vi "DI Read_v1.vi"(8 "error in (no error)":errorcluster, 11 "ControlBoard VISA":refnum<visa-resource-name>="ControlBoard") -> (0 "error out":errorcluster, 1 "DI Reading (Hex String)":string, 2 "DI Reading":bool[](array[boolean]), 3 "VISA Refnum out":refnum<visa-resource-name>)   [LabVIEW 2019]
uses:
  <vilib>/Instr/_visa.llb/VISA Flush IO Buffer Mask.ctl
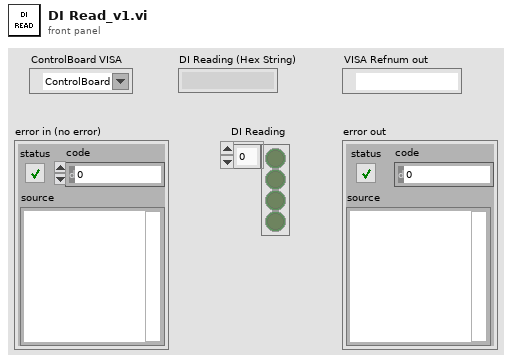
[diagram p1: front panel]
types:
  T1 = typedef "VISA Flush IO Buffer Mask.ctl" = u16
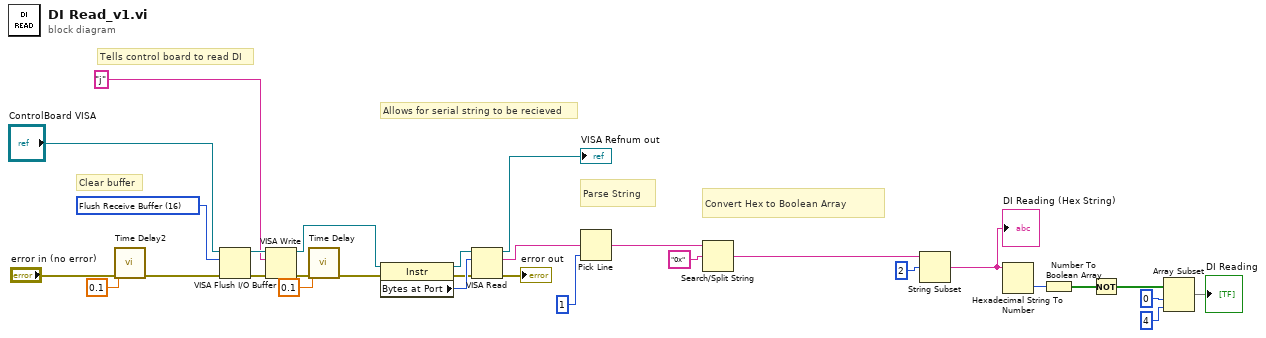
[diagram p0: block diagram]
diagram:
  w19 = T1 16 items=["Flush Receive Buffer"=16, "Write Transmit Buffer to Device"=32, "Flush Receive Buffer (No I/O)"=64, "Flush Transmit Buffer"=128] ("Mask")
  # "Convert Hex to Boolean Array"
  # "Clear buffer"
  # "Parse String"
  # "Allows for serial string to be recieved"
  # "Tells control board to read DI"
  n1 = call "Time Delay2"("error in (no error)"="error in (no error)", "Delay Time (s)"=0.1) -> ("error out"=w5:errorcluster)  [unwired: 9 in]
  n2 = VISA Flush I/O Buffer(VISA resource name="ControlBoard VISA", mask (16)=w19, error in (no error)=w5) -> (VISA resource name out=w21:refnum<visa-resource-name>, error out=w22:errorcluster)
  n3 = VISA Write(VISA resource name=w21, write buffer="j", error in (no error)=w22) -> (VISA resource name out=w24:refnum<visa-resource-name>, error out=w20:errorcluster)  [unwired: 1 out]
  n4 = call "Time Delay"("error in (no error)"=w20, "Delay Time (s)"=0.1) -> ("error out"=w23:errorcluster)  [unwired: 9 in]
  n5 = property class="Instr"(reference=w24, error in=w23) -> (reference out=w16:refnum<visa-resource-name>, error out=w17:errorcluster, "Bytes at Port"=w18:u32)
  n6 = VISA Read(VISA resource name=w16, byte count=w18, error in (no error)=w17) -> (VISA resource name out=→"VISA Refnum out":refnum<visa-resource-name>, read buffer=w28:string, error out=→"error out":errorcluster)  [unwired: 1 out]
  n7 = Pick Line(multi-line string=w28, line index=1) -> (output string=w29:string)  [unwired: 1 in]
  n8 = Search/Split String(string=w29, search string/char (-)="0x" ("regular expression")) -> (match + rest of string=w26:string)  [unwired: 1 in, 2 out]
  n9 = String Subset(string=w26, offset (0)=2) -> (substring=w10:string)  [unwired: 1 in]
  "DI Reading (Hex String)" <- w10
  n10 = Hexadecimal String To Number(string=w10) -> (number=w12:u32)  [unwired: 2 in, 1 out]
  n11 = Number To Boolean Array(number=w12) -> (Boolean array=w11:bool[])
  n12 = Not(x=w11) -> (.not. x?=w7:bool[])
  n13 = Array Subset(array=w7, index=0, length=4) -> (→"DI Reading":bool[])
